vi "Binary search.vi"(8 "element":u64, 11 "1D array":u64[](array[numeric])) -> (3 "index":i32)   [LabVIEW 2016]
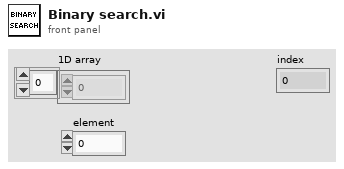
[diagram p1: front panel]
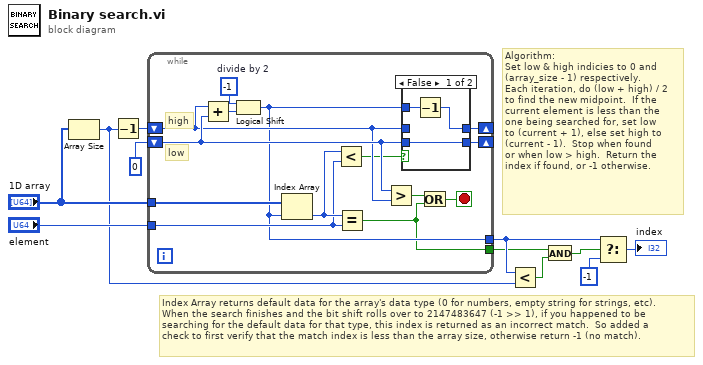
[diagram p0: block diagram]
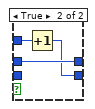
[diagram p2: hidden frame]
diagram:
  # "Index Array returns default data for the array's data type (0 for numbers, empty string for strings, etc).\nWhen the search finishes and the bit shift rolls over to 2147483647 (-1 >> 1), if you happened to be\nsearching for the default data for that type, this index is returned as an incorrect match.  So added a\ncheck to first verify that the match index is less than the array size, otherwise return -1 (no match)."
  # "Algorithm:\nSet low & high indicies to 0 and\n(array_size - 1) respectively.\nEach iteration, do (low + high) / 2\nto find the new midpoint.  If the\ncurrent element is less than the\none being searched for, set low\nto (current + 1), else set high to\n(current - 1).  Stop when found\nor when low > high.  Return the\nindex if found, or -1 otherwise."
  n1 = Array Size(array="1D array") -> (size(s)=w2:i32)
  n2 = Decrement(x=w2) -> (x-1=w8:i32)
  n3 = while {
    tunnel: "1D array" -> [w25]
    tunnel: "element" -> [w20]
    shift-right: [w19] -> _
    shift-left: w8 -> [w16]
    tunnel: [w12] -> w1
    shift-right: [w18] -> _
    shift-left: 0 -> [w17]
    tunnel: [w14] -> w3
    stop <- w24 stop-if-true
    w22 = -1  # divide by 2
    # "low"
    # "high"
    n4 = Add(x=w16, y=w17) -> (x+y=w23:i32)
    n5 = Logical Shift(y=w22, x=w23) -> (x << y=w14:i32)
    n6 = Index Array(array=w25, index=w14) -> (element=w21:u64)
    n7 = Less?(x=w21, y=w20) -> (x < y?=w15:bool)
    n8 = Equal?(x=w21, y=w20) -> (x = y?=w12:bool)
    n9 = Greater?(x=w17, y=w16) -> (0:w13:bool)
    n10 = case shown="False" w15 {
      tunnel: w16 -> [_ w31]
      tunnel: w17 -> [w27 _]
      tunnel: [w26 w31] -> w19
      tunnel: w14 -> [w28 w30]
      tunnel: [w27 w29] -> w18
      frame False {
        n11 = Decrement(x=w28) -> (x-1=w26:i32)
      }
      frame True {
        n12 = Increment(x=w30) -> (x+1=w29:i32)
      }
    }
    n13 = Or(x=w13, y=w12) -> (x .or. y?=w24:bool)
  }
  n14 = Less?(x=w3, y=w2) -> (x < y?=w5:bool)
  n15 = And(x=w1, y=w5) -> (x .and. y?=w4:bool)
  n16 = Select(t=w3, s=w4, f=-1) -> (s? t:f=→"index":i32)
